vi "adp.vi"() -> ()   [LabVIEW 2020]
panel:
  in  "new element/subarray":dbl
  in  "index":i32
  out "output array":dbl[](array[numeric])
  out "Waveform Graph":dynamicdata(graph)
  in  "stop":bool
  out "Array":dbl[](array[numeric])
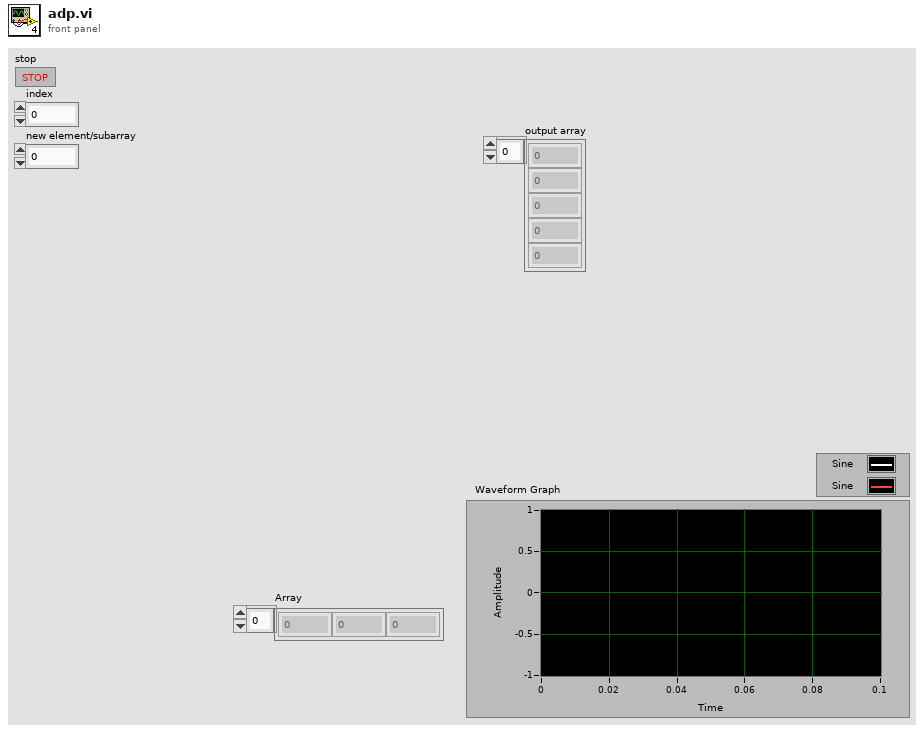
[diagram p1: front panel]
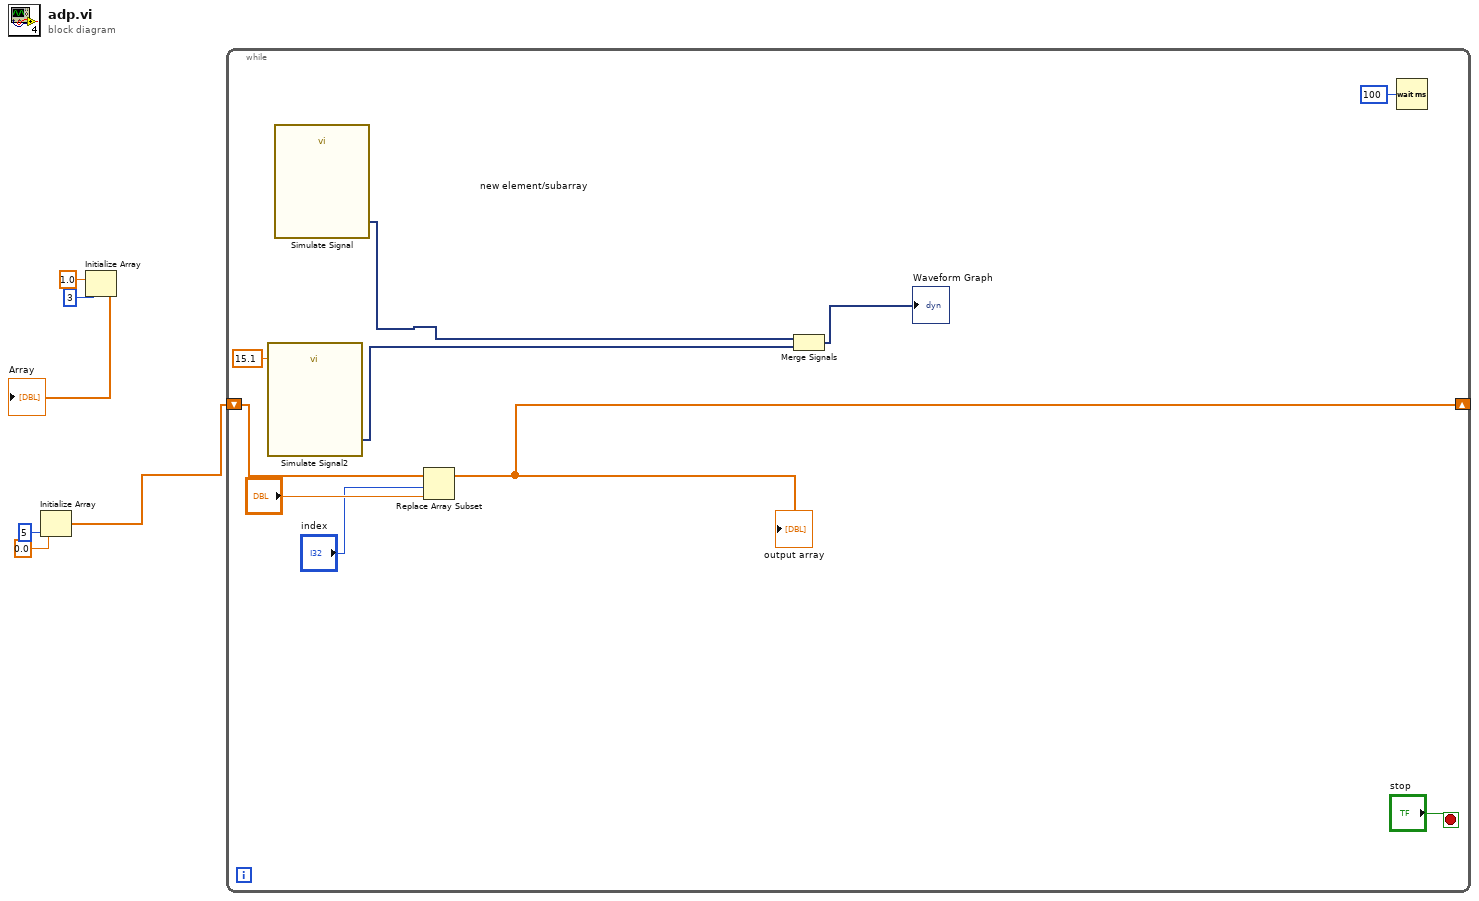
[diagram p0: block diagram]
diagram:
  n1 = Initialize Array(0.0 ("element"), 5 ("dimension size")) -> (w3:dbl[])
  n2 = Initialize Array(1.0 ("element"), 3 ("dimension size")) -> (→"Array":dbl[])
  n3 = while {
    shift-right: [w8] -> _
    shift-left: w3 -> [w7]
    stop <- "stop" stop-if-true
    n4 = call "Simulate Signal2"("Frequency"=15.1) -> ("Sine"=w13:dynamicdata)  [unwired: 13 in, 1 out]
    n5 = call "Simulate Signal"() -> ("Sine"=w14:dynamicdata)  [unwired: 14 in, 1 out]
    n6 = Replace Array Subset(array=w7, new element="new element/subarray", index="index") -> (w8:dbl[])
    "output array" <- w8
    n7 = Merge Signals(w14, w13) -> (→"Waveform Graph":dynamicdata)
    n8 = Wait (ms)(milliseconds to wait=u32 100) -> ()  [unwired: 1 out]
  }
